vi "Estado-IPS.vi"(2 "VISA resource name":refnum<visa-resource-name>="COM1") -> (0 "read string":string)   [LabVIEW 2011]
doc: "The Advanced Serial Read and Write example performs a Serial Port Read, a Serial Port Write, or a combination of these actions while setting some advanced serial features like buffer size, termination characters, and XON/XOFF flow control. The user selects the actions (read or write) on the front panel. If both are selected, the VI will write the data first, read the data and then close the VISA session that is opened to the port. \n\nThe parameters set for the serial port must match the parameters of the connected instrument or device. In this example, the bytes to read parameter specifies the number of bytes that the serial port reads. If there were more bytes at the port than the number specified in bytes to read, those bytes would not be read. Also, if you specify to read more bytes than the number of bytes actually read, you might receive a timeout error message.\n\nINSTRUCTIONS:\n1) Select the serial resource and configuration parameters (baud rate, data bits, parity, stop bits, flow control).\n2) Termination character can be enabled and set. Also, set the required input buffer size prior to running the example.\n3) Select the operations to be performed. \n4) Connect the serial port to your device. If no device is available, perform a loopback test by doing one of the following. Short pins 2 and 3 on a RS-232 cable or short pin 4 to pin 8 and pin 5 to pin 9 on a RS-485/422 cable. \n5) Run the VI to see the data read. (The \"read string\" will match the \"string to write\" if a loopback test was performed.)\n\nThis example exposes several advanced features that you may need for your application. Not all applications need all the features shown in this example. The input buffer size is likely an important setting that you want to control in your application. This example expands upon the flow control option for XON and XOFF, allowing the user to choose those control characters. The timeout parameter has been brought to the front panel so a user can specify the time period the VISA Read will wait for the number of bytes to read before timing out. Also, the user has several controls for the termination character, which is discussed later.\n\nNote that you can press the write and read buttons and change the bytes to read parameters on the fly, while the example is running. However, you must stop the example to change the other configuration parameters after the example has started running, and then run again.\n\nSet the I/O buffer size slightly higher the amount of data you expect to receive. This is very important for applications that don't use flow control, as you may lose characters if the receive buffer overflows.\n\nSetting the timeout period ensures that the operation returns with a timeout error if the operation cannot be performed in the specified time period. \n\nSome devices require a termination character in order to identify the end of command strings. Some devices send a termination character to signify the end of data to be read. \n\nThis example shows how you can end the Read operation once a termination character is detected in the buffer and/or append a termination character at the end of the Write data. To enable the Read to end on a termination character, use the VISA Configure Serial Port or use the VISA Properties Serial End Mode for Reads, Termination Character Enable, and Termination Character. To end the Write with a termination character, use the VISA Properties Serial End Mode for Writes, the Send End Enable, and Termination Character. In this example, the same termination character is used for both the Read and the Write. You can specify two different characters for your application, if desired.\n\nYour application may require specific characters for the XON/XOFF Flow Control. You can specify these characters with the VISA Properties Flow Control XOFF Character and Flow Control XON Character. Note that if the standard XON and XOFF characters are used, then decimal 17 and 19 are unavailable for data values. Remember that using flow control and setting an adequate buffer size allow you to prevent buffer overflows."
uses:
  <vilib>/Instr/_visa.llb/VISA Configure Serial Port (Instr).vi
panel:
  out "read string 2":string
  out "actual bytes read":u32
  in  "read":bool=TRUE
  in  "bytes to read":u32=1000
  in  "flow control":u16(ring) items=["None"=0, "XON/XOFF"=1, "RTS/CTS"=2, "DTR/DSR"=4]
  in  "End write with termination character?":bool=TRUE
  in  "Input\nbuffer size":u32=4096
  in  "termination char\n(0xA = '\\n' = LF)":u8=13 format="%.0x"
  in  "End read on termination character?":bool=TRUE
  in  "timeout (ms)":u32=10000
  in  "parity":u16(ring) items=["None", "Odd", "Even", "Mark", "Space"]
  in  "data bits":u16=8 min=5 max=8 step=1
  in  "stop bits":u16(ring)=10 items=["1.0"=10, "1.5"=15, "2.0"=20]
  in  "baud rate":u32=2400
  in  "write":bool=TRUE
  in  "string to write":string="L"
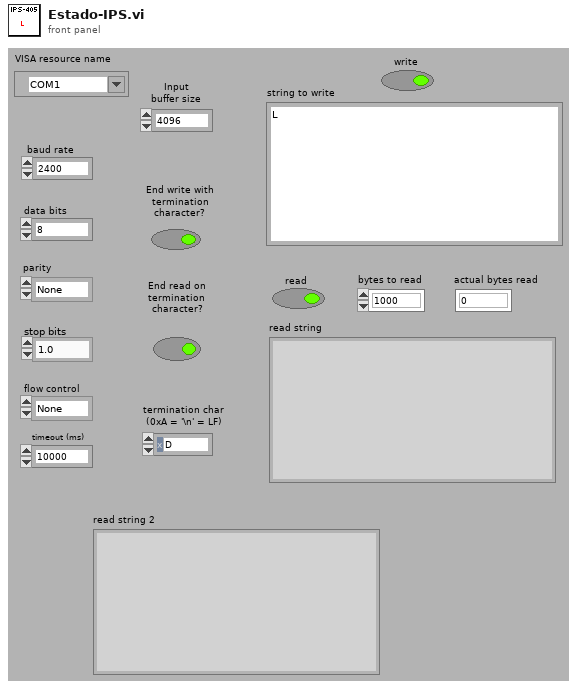
[diagram p1: front panel]
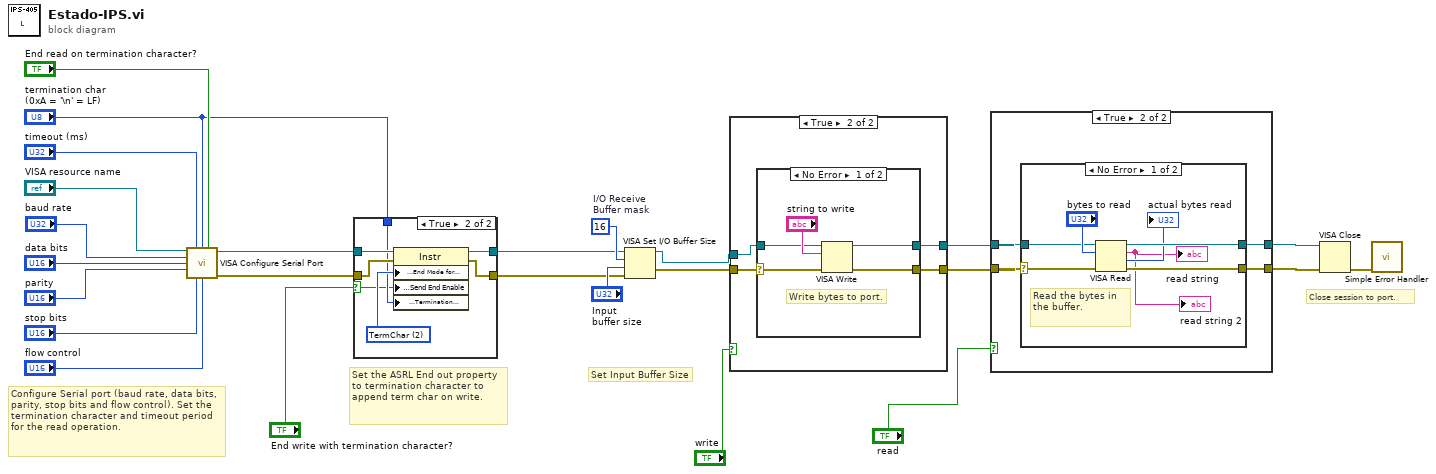
[diagram p0: block diagram]
diagram:
  w18 = u16 16  # I/O Receive Buffer mask
  # "Configure Serial port (baud rate, data bits, parity, stop bits and flow control). Set the termination character and timeout period for the read operation."
  # "Set Input Buffer Size"
  # "Set the ASRL End out property to termination character to append term char on write."
  # "Close session to port."
  n1 = call-poly "VISA Configure Serial Port"("VISA resource name"="VISA resource name", "timeout (10sec)"="timeout (ms)", "termination char\n(0xA = '\\n' = LF)"="termination char\n(0xA = '\\n' = LF)", "Enable Termination\nChar (T)"="End read on termination character?", "baud rate (9600)"="baud rate", "data bits (8)"="data bits", "parity (0:none)"="parity", "stop bits (10: 1 bit)"="stop bits", "flow control (0:none)"="flow control") -> ("VISA resource name out"=w9:refnum<visa-resource-name>, "error out"=w12:errorcluster)  [unwired: 1 in, 4 out]
  n2 = case shown="True" "End write with termination character?" {
    selector: "End write with termination character?" -> [_ w28]
    tunnel: w9 -> [w26 w34]
    tunnel: w12 -> [w27 w33]
    tunnel: [w26 w32] -> w10
    tunnel: [w27 w31] -> w11
    tunnel: "termination char\n(0xA = '\\n' = LF)" -> [_ w29]
    frame False {
    }
    frame True {
      w30 = u16 2 items=["None", "LastBit", "TermChar", "Break"] ("Serial Settings:Serial End Mode for Writes")
      n3 = property class="Instr"(reference=w34, error in=w33, "Serial Settings:End Mode for Writes"=w30, "Message Based Settings:Send End Enable"=w28, "Message Based Settings:Termination Character"=w29) -> (reference out=w32:refnum<visa-resource-name>, error out=w31:errorcluster)
    }
  }
  n4 = VISA Set I/O Buffer Size(VISA resource name=w10, mask (16)=w18, size (4096)="Input\nbuffer size", error in (no error)=w11) -> (VISA resource name out=w2:refnum<visa-resource-name>, error out=w1:errorcluster)
  n5 = case shown="True" "write" {
    tunnel: [w35 w40] -> w6
    tunnel: [w36 w39] -> w7
    tunnel: w1 -> [w36 w37]
    tunnel: w2 -> [w35 w38]
    frame False {
    }
    frame True {
      n6 = case shown="No Error" w37 {
        selector: w37 -> [w42 w47]
        tunnel: [w45 w46] -> w40
        tunnel: [w44 w47] -> w39
        tunnel: w38 -> [w41 w46]
        frame No Error {
          # "Write bytes to port."
          n7 = VISA Write(VISA resource name=w41, write buffer="string to write", error in (no error)=w42) -> (VISA resource name out=w45:refnum<visa-resource-name>, error out=w44:errorcluster)  [unwired: 1 out]
        }
        frame Error {
        }
      }
    }
  }
  n8 = case shown="True" "read" {
    tunnel: w7 -> [w48 w51]
    tunnel: w6 -> [w49 w50]
    tunnel: [w48 w53] -> w3
    tunnel: [w49 w52] -> w4
    frame False {
    }
    frame True {
      n9 = case "Read bytes from port." shown="No Error" w51 {
        selector: w51 -> [w56 w61]
        tunnel: [w59 w61] -> w53
        tunnel: [w60 w62] -> w52
        tunnel: w50 -> [w57 w62]
        frame No Error {
          # "Read the bytes in the buffer."
          n10 = VISA Read(VISA resource name=w57, byte count="bytes to read", error in (no error)=w56) -> (VISA resource name out=w60:refnum<visa-resource-name>, read buffer=→"read string" →"read string 2":string, return count=→"actual bytes read":u32, error out=w59:errorcluster)
        }
        frame Error {
          # "Error occurred \nreading Bytes at \nSerial Port"
        }
      }
    }
  }
  n11 = VISA Close(VISA resource name=w4, error in (no error)=w3) -> (error out=w23:errorcluster)
  n12 = call <vilib>:"Simple Error Handler.vi"("error in (no error)"=w23) -> ()  [unwired: 1 in, 8 out]
